vi "Main.vi"() -> ()   [LabVIEW 2021] (continued)
                w86 = T9 27 items=["刷新间隔", "波特率", "布尔1设置项", "布尔2设置项", "布尔3设置项", "布尔4设置项", "布尔5设置项", "布尔6设置项", "布尔7设置项", "布尔8设置项", "显控1设置", "显控2设置", "显控3设置", "显控4设置", "显控5设置", "显控6设置", "显控7设置", "显控8设置", "显控9设置", "显控10设置", "显控11设置", "显控12设置", "设控1设置", "设控2设置", "设控3设置", "设控4设置", "设控5设置", "设控6设置", "设控7设置", "设控8设置", "曲线1设置", "曲线2设置", "曲线3设置", "曲线4设置", "曲线5设置", "曲线6设置", "曲线7设置", "曲线8设置", "曲线9设置", "曲线10设置", "曲线11设置", "曲线12设置", "曲线13设置", "曲线14设置", "曲线15设置", "曲线16设置", "曲线17设置", "曲线18设置", "曲线19设置", "曲线20设置", "曲线21设置", "曲线22设置", "曲线23设置", "曲线24设置", "曲线25设置", "曲线26设置", "曲线27设置", "曲线28设置", "曲线29设置", "曲线30设置", "曲线31设置", "曲线32设置", "曲线33设置", "曲线34设置", "曲线35设置", "曲线36设置", "曲线37设置", "曲线38设置", "曲线39设置", "曲线40设置", "曲线41设置", "曲线42设置", "曲线43设置", "曲线44设置", "曲线45设置", "曲线46设置", "曲线47设置", "曲线48设置", "曲线49设置", "曲线50设置", "曲线51设置", "曲线52设置", "曲线53设置", "曲线54设置", "曲线55设置", "曲线56设置", "曲线57设置", "曲线58设置", "曲线59设置", "曲线60设置", "曲线61设置", "曲线62设置", "曲线63设置", "曲线64设置", "ID值", "数据模式"] ("DataInitDef")
                w87 = T9 26 items=["刷新间隔", "波特率", "布尔1设置项", "布尔2设置项", "布尔3设置项", "布尔4设置项", "布尔5设置项", "布尔6设置项", "布尔7设置项", "布尔8设置项", "显控1设置", "显控2设置", "显控3设置", "显控4设置", "显控5设置", "显控6设置", "显控7设置", "显控8设置", "显控9设置", "显控10设置", "显控11设置", "显控12设置", "设控1设置", "设控2设置", "设控3设置", "设控4设置", "设控5设置", "设控6设置", "设控7设置", "设控8设置", "曲线1设置", "曲线2设置", "曲线3设置", "曲线4设置", "曲线5设置", "曲线6设置", "曲线7设置", "曲线8设置", "曲线9设置", "曲线10设置", "曲线11设置", "曲线12设置", "曲线13设置", "曲线14设置", "曲线15设置", "曲线16设置", "曲线17设置", "曲线18设置", "曲线19设置", "曲线20设置", "曲线21设置", "曲线22设置", "曲线23设置", "曲线24设置", "曲线25设置", "曲线26设置", "曲线27设置", "曲线28设置", "曲线29设置", "曲线30设置", "曲线31设置", "曲线32设置", "曲线33设置", "曲线34设置", "曲线35设置", "曲线36设置", "曲线37设置", "曲线38设置", "曲线39设置", "曲线40设置", "曲线41设置", "曲线42设置", "曲线43设置", "曲线44设置", "曲线45设置", "曲线46设置", "曲线47设置", "曲线48设置", "曲线49设置", "曲线50设置", "曲线51设置", "曲线52设置", "曲线53设置", "曲线54设置", "曲线55设置", "曲线56设置", "曲线57设置", "曲线58设置", "曲线59设置", "曲线60设置", "曲线61设置", "曲线62设置", "曲线63设置", "曲线64设置", "ID值", "数据模式"] ("DataInitDef")
                w88 = T9 29 items=["刷新间隔", "波特率", "布尔1设置项", "布尔2设置项", "布尔3设置项", "布尔4设置项", "布尔5设置项", "布尔6设置项", "布尔7设置项", "布尔8设置项", "显控1设置", "显控2设置", "显控3设置", "显控4设置", "显控5设置", "显控6设置", "显控7设置", "显控8设置", "显控9设置", "显控10设置", "显控11设置", "显控12设置", "设控1设置", "设控2设置", "设控3设置", "设控4设置", "设控5设置", "设控6设置", "设控7设置", "设控8设置", "曲线1设置", "曲线2设置", "曲线3设置", "曲线4设置", "曲线5设置", "曲线6设置", "曲线7设置", "曲线8设置", "曲线9设置", "曲线10设置", "曲线11设置", "曲线12设置", "曲线13设置", "曲线14设置", "曲线15设置", "曲线16设置", "曲线17设置", "曲线18设置", "曲线19设置", "曲线20设置", "曲线21设置", "曲线22设置", "曲线23设置", "曲线24设置", "曲线25设置", "曲线26设置", "曲线27设置", "曲线28设置", "曲线29设置", "曲线30设置", "曲线31设置", "曲线32设置", "曲线33设置", "曲线34设置", "曲线35设置", "曲线36设置", "曲线37设置", "曲线38设置", "曲线39设置", "曲线40设置", "曲线41设置", "曲线42设置", "曲线43设置", "曲线44设置", "曲线45设置", "曲线46设置", "曲线47设置", "曲线48设置", "曲线49设置", "曲线50设置", "曲线51设置", "曲线52设置", "曲线53设置", "曲线54设置", "曲线55设置", "曲线56设置", "曲线57设置", "曲线58设置", "曲线59设置", "曲线60设置", "曲线61设置", "曲线62设置", "曲线63设置", "曲线64设置", "ID值", "数据模式"] ("DataInitDef")
                w89 = T9 24 items=["刷新间隔", "波特率", "布尔1设置项", "布尔2设置项", "布尔3设置项", "布尔4设置项", "布尔5设置项", "布尔6设置项", "布尔7设置项", "布尔8设置项", "显控1设置", "显控2设置", "显控3设置", "显控4设置", "显控5设置", "显控6设置", "显控7设置", "显控8设置", "显控9设置", "显控10设置", "显控11设置", "显控12设置", "设控1设置", "设控2设置", "设控3设置", "设控4设置", "设控5设置", "设控6设置", "设控7设置", "设控8设置", "曲线1设置", "曲线2设置", "曲线3设置", "曲线4设置", "曲线5设置", "曲线6设置", "曲线7设置", "曲线8设置", "曲线9设置", "曲线10设置", "曲线11设置", "曲线12设置", "曲线13设置", "曲线14设置", "曲线15设置", "曲线16设置", "曲线17设置", "曲线18设置", "曲线19设置", "曲线20设置", "曲线21设置", "曲线22设置", "曲线23设置", "曲线24设置", "曲线25设置", "曲线26设置", "曲线27设置", "曲线28设置", "曲线29设置", "曲线30设置", "曲线31设置", "曲线32设置", "曲线33设置", "曲线34设置", "曲线35设置", "曲线36设置", "曲线37设置", "曲线38设置", "曲线39设置", "曲线40设置", "曲线41设置", "曲线42设置", "曲线43设置", "曲线44设置", "曲线45设置", "曲线46设置", "曲线47设置", "曲线48设置", "曲线49设置", "曲线50设置", "曲线51设置", "曲线52设置", "曲线53设置", "曲线54设置", "曲线55设置", "曲线56设置", "曲线57设置", "曲线58设置", "曲线59设置", "曲线60设置", "曲线61设置", "曲线62设置", "曲线63设置", "曲线64设置", "ID值", "数据模式"] ("DataInitDef")
                w90 = T9 25 items=["刷新间隔", "波特率", "布尔1设置项", "布尔2设置项", "布尔3设置项", "布尔4设置项", "布尔5设置项", "布尔6设置项", "布尔7设置项", "布尔8设置项", "显控1设置", "显控2设置", "显控3设置", "显控4设置", "显控5设置", "显控6设置", "显控7设置", "显控8设置", "显控9设置", "显控10设置", "显控11设置", "显控12设置", "设控1设置", "设控2设置", "设控3设置", "设控4设置", "设控5设置", "设控6设置", "设控7设置", "设控8设置", "曲线1设置", "曲线2设置", "曲线3设置", "曲线4设置", "曲线5设置", "曲线6设置", "曲线7设置", "曲线8设置", "曲线9设置", "曲线10设置", "曲线11设置", "曲线12设置", "曲线13设置", "曲线14设置", "曲线15设置", "曲线16设置", "曲线17设置", "曲线18设置", "曲线19设置", "曲线20设置", "曲线21设置", "曲线22设置", "曲线23设置", "曲线24设置", "曲线25设置", "曲线26设置", "曲线27设置", "曲线28设置", "曲线29设置", "曲线30设置", "曲线31设置", "曲线32设置", "曲线33设置", "曲线34设置", "曲线35设置", "曲线36设置", "曲线37设置", "曲线38设置", "曲线39设置", "曲线40设置", "曲线41设置", "曲线42设置", "曲线43设置", "曲线44设置", "曲线45设置", "曲线46设置", "曲线47设置", "曲线48设置", "曲线49设置", "曲线50设置", "曲线51设置", "曲线52设置", "曲线53设置", "曲线54设置", "曲线55设置", "曲线56设置", "曲线57设置", "曲线58设置", "曲线59设置", "曲线60设置", "曲线61设置", "曲线62设置", "曲线63设置", "曲线64设置", "ID值", "数据模式"] ("DataInitDef")
                w91 = T9 23 items=["刷新间隔", "波特率", "布尔1设置项", "布尔2设置项", "布尔3设置项", "布尔4设置项", "布尔5设置项", "布尔6设置项", "布尔7设置项", "布尔8设置项", "显控1设置", "显控2设置", "显控3设置", "显控4设置", "显控5设置", "显控6设置", "显控7设置", "显控8设置", "显控9设置", "显控10设置", "显控11设置", "显控12设置", "设控1设置", "设控2设置", "设控3设置", "设控4设置", "设控5设置", "设控6设置", "设控7设置", "设控8设置", "曲线1设置", "曲线2设置", "曲线3设置", "曲线4设置", "曲线5设置", "曲线6设置", "曲线7设置", "曲线8设置", "曲线9设置", "曲线10设置", "曲线11设置", "曲线12设置", "曲线13设置", "曲线14设置", "曲线15设置", "曲线16设置", "曲线17设置", "曲线18设置", "曲线19设置", "曲线20设置", "曲线21设置", "曲线22设置", "曲线23设置", "曲线24设置", "曲线25设置", "曲线26设置", "曲线27设置", "曲线28设置", "曲线29设置", "曲线30设置", "曲线31设置", "曲线32设置", "曲线33设置", "曲线34设置", "曲线35设置", "曲线36设置", "曲线37设置", "曲线38设置", "曲线39设置", "曲线40设置", "曲线41设置", "曲线42设置", "曲线43设置", "曲线44设置", "曲线45设置", "曲线46设置", "曲线47设置", "曲线48设置", "曲线49设置", "曲线50设置", "曲线51设置", "曲线52设置", "曲线53设置", "曲线54设置", "曲线55设置", "曲线56设置", "曲线57设置", "曲线58设置", "曲线59设置", "曲线60设置", "曲线61设置", "曲线62设置", "曲线63设置", "曲线64设置", "ID值", "数据模式"] ("DataInitDef")
                w92 = T9 94 items=["刷新间隔", "波特率", "布尔1设置项", "布尔2设置项", "布尔3设置项", "布尔4设置项", "布尔5设置项", "布尔6设置项", "布尔7设置项", "布尔8设置项", "显控1设置", "显控2设置", "显控3设置", "显控4设置", "显控5设置", "显控6设置", "显控7设置", "显控8设置", "显控9设置", "显控10设置", "显控11设置", "显控12设置", "设控1设置", "设控2设置", "设控3设置", "设控4设置", "设控5设置", "设控6设置", "设控7设置", "设控8设置", "曲线1设置", "曲线2设置", "曲线3设置", "曲线4设置", "曲线5设置", "曲线6设置", "曲线7设置", "曲线8设置", "曲线9设置", "曲线10设置", "曲线11设置", "曲线12设置", "曲线13设置", "曲线14设置", "曲线15设置", "曲线16设置", "曲线17设置", "曲线18设置", "曲线19设置", "曲线20设置", "曲线21设置", "曲线22设置", "曲线23设置", "曲线24设置", "曲线25设置", "曲线26设置", "曲线27设置", "曲线28设置", "曲线29设置", "曲线30设置", "曲线31设置", "曲线32设置", "曲线33设置", "曲线34设置", "曲线35设置", "曲线36设置", "曲线37设置", "曲线38设置", "曲线39设置", "曲线40设置", "曲线41设置", "曲线42设置", "曲线43设置", "曲线44设置", "曲线45设置", "曲线46设置", "曲线47设置", "曲线48设置", "曲线49设置", "曲线50设置", "曲线51设置", "曲线52设置", "曲线53设置", "曲线54设置", "曲线55设置", "曲线56设置", "曲线57设置", "曲线58设置", "曲线59设置", "曲线60设置", "曲线61设置", "曲线62设置", "曲线63设置", "曲线64设置", "ID值", "数据模式"] ("DataInitDef")
                w93 = T9 22 items=["刷新间隔", "波特率", "布尔1设置项", "布尔2设置项", "布尔3设置项", "布尔4设置项", "布尔5设置项", "布尔6设置项", "布尔7设置项", "布尔8设置项", "显控1设置", "显控2设置", "显控3设置", "显控4设置", "显控5设置", "显控6设置", "显控7设置", "显控8设置", "显控9设置", "显控10设置", "显控11设置", "显控12设置", "设控1设置", "设控2设置", "设控3设置", "设控4设置", "设控5设置", "设控6设置", "设控7设置", "设控8设置", "曲线1设置", "曲线2设置", "曲线3设置", "曲线4设置", "曲线5设置", "曲线6设置", "曲线7设置", "曲线8设置", "曲线9设置", "曲线10设置", "曲线11设置", "曲线12设置", "曲线13设置", "曲线14设置", "曲线15设置", "曲线16设置", "曲线17设置", "曲线18设置", "曲线19设置", "曲线20设置", "曲线21设置", "曲线22设置", "曲线23设置", "曲线24设置", "曲线25设置", "曲线26设置", "曲线27设置", "曲线28设置", "曲线29设置", "曲线30设置", "曲线31设置", "曲线32设置", "曲线33设置", "曲线34设置", "曲线35设置", "曲线36设置", "曲线37设置", "曲线38设置", "曲线39设置", "曲线40设置", "曲线41设置", "曲线42设置", "曲线43设置", "曲线44设置", "曲线45设置", "曲线46设置", "曲线47设置", "曲线48设置", "曲线49设置", "曲线50设置", "曲线51设置", "曲线52设置", "曲线53设置", "曲线54设置", "曲线55设置", "曲线56设置", "曲线57设置", "曲线58设置", "曲线59设置", "曲线60设置", "曲线61设置", "曲线62设置", "曲线63设置", "曲线64设置", "ID值", "数据模式"] ("DataInitDef")
                w103 = 0 ("禁用的索引 (列)")
                w102 = 0 ("禁用的索引 (列)")
                n54 = local read "控件配置文件"() -> (w96:string[][])
                n55 = local read "控件配置文件"() -> (w108:string[][])
                n56 = Index Array(array=w96, index (row)=w93, index (col)=w102) -> (element=w111:string)
                n57 = Index Array(array=w96, index (row)=w91, index (col)=w102) -> (element=w110:string)
                n58 = Index Array(array=w96, index (row)=w90, index (col)=w102) -> (element=w109:string)
                n59 = Index Array(array=w96, index (row)=w89, index (col)=w102) -> (element=w112:string)
                n60 = Index Array(array=w108, index (row)=w88, index (col)=w103) -> (element=w107:string)
                n61 = Index Array(array=w108, index (row)=w87, index (col)=w103) -> (element=w105:string)
                n62 = Index Array(array=w108, index (row)=w86, index (col)=w103) -> (element=w106:string)
                n63 = Index Array(array=w108, index (row)=w85, index (col)=w103) -> (element=w104:string)
                n64 = Index Array(array=w96, index (row)=w92, index (col)=1 ("禁用的索引 (列)")) -> (element=w100:string)
                n65 = property on="设控1" class="Str"("Caption.Text"=w111) -> ()  [unwired: 2 in, 2 out]
                n66 = property on="设控2" class="Str"("Caption.Text"=w110) -> ()  [unwired: 2 in, 2 out]
                n67 = property on="设控4" class="Str"("Caption.Text"=w109) -> ()  [unwired: 2 in, 2 out]
                n68 = property on="设控3" class="Str"("Caption.Text"=w112) -> ()  [unwired: 2 in, 2 out]
                n69 = property on="设控8" class="Str"("Caption.Text"=w107) -> ()  [unwired: 2 in, 2 out]
                n70 = property on="设控5" class="Str"("Caption.Text"=w105) -> ()  [unwired: 2 in, 2 out]
                n71 = property on="设控6" class="Str"("Caption.Text"=w106) -> ()  [unwired: 2 in, 2 out]
                n72 = property on="设控7" class="Str"("Caption.Text"=w104) -> ()  [unwired: 2 in, 2 out]
                n73 = Hexadecimal String To Number(string=w100) -> (number=w99:u32)  [unwired: 2 in, 1 out]
                n74 = local write "ID"(w99) -> ()
                n75 = Index Array(array=w96, index (row)=w84, index (col)=1 ("禁用的索引 (列)")) -> (element=w97:string)
                n76 = Hexadecimal String To Number(string=w97) -> (number=w95:u32)  [unwired: 2 in, 1 out]
                n77 = Not Equal To 0?(x=w95) -> (x != 0?=w94:bool)
                n78 = local write "数据模式"(w94) -> ()
              }
              frame #3 {
                w113 = T9 9 items=["刷新间隔", "波特率", "布尔1设置项", "布尔2设置项", "布尔3设置项", "布尔4设置项", "布尔5设置项", "布尔6设置项", "布尔7设置项", "布尔8设置项", "显控1设置", "显控2设置", "显控3设置", "显控4设置", "显控5设置", "显控6设置", "显控7设置", "显控8设置", "显控9设置", "显控10设置", "显控11设置", "显控12设置", "设控1设置", "设控2设置", "设控3设置", "设控4设置", "设控5设置", "设控6设置", "设控7设置", "设控8设置", "曲线1设置", "曲线2设置", "曲线3设置", "曲线4设置", "曲线5设置", "曲线6设置", "曲线7设置", "曲线8设置", "曲线9设置", "曲线10设置", "曲线11设置", "曲线12设置", "曲线13设置", "曲线14设置", "曲线15设置", "曲线16设置", "曲线17设置", "曲线18设置", "曲线19设置", "曲线20设置", "曲线21设置", "曲线22设置", "曲线23设置", "曲线24设置", "曲线25设置", "曲线26设置", "曲线27设置", "曲线28设置", "曲线29设置", "曲线30设置", "曲线31设置", "曲线32设置", "曲线33设置", "曲线34设置", "曲线35设置", "曲线36设置", "曲线37设置", "曲线38设置", "曲线39设置", "曲线40设置", "曲线41设置", "曲线42设置", "曲线43设置", "曲线44设置", "曲线45设置", "曲线46设置", "曲线47设置", "曲线48设置", "曲线49设置", "曲线50设置", "曲线51设置", "曲线52设置", "曲线53设置", "曲线54设置", "曲线55设置", "曲线56设置", "曲线57设置", "曲线58设置", "曲线59设置", "曲线60设置", "曲线61设置", "曲线62设置", "曲线63设置", "曲线64设置", "ID值", "数据模式"] ("DataInitDef")
                w114 = T9 8 items=["刷新间隔", "波特率", "布尔1设置项", "布尔2设置项", "布尔3设置项", "布尔4设置项", "布尔5设置项", "布尔6设置项", "布尔7设置项", "布尔8设置项", "显控1设置", "显控2设置", "显控3设置", "显控4设置", "显控5设置", "显控6设置", "显控7设置", "显控8设置", "显控9设置", "显控10设置", "显控11设置", "显控12设置", "设控1设置", "设控2设置", "设控3设置", "设控4设置", "设控5设置", "设控6设置", "设控7设置", "设控8设置", "曲线1设置", "曲线2设置", "曲线3设置", "曲线4设置", "曲线5设置", "曲线6设置", "曲线7设置", "曲线8设置", "曲线9设置", "曲线10设置", "曲线11设置", "曲线12设置", "曲线13设置", "曲线14设置", "曲线15设置", "曲线16设置", "曲线17设置", "曲线18设置", "曲线19设置", "曲线20设置", "曲线21设置", "曲线22设置", "曲线23设置", "曲线24设置", "曲线25设置", "曲线26设置", "曲线27设置", "曲线28设置", "曲线29设置", "曲线30设置", "曲线31设置", "曲线32设置", "曲线33设置", "曲线34设置", "曲线35设置", "曲线36设置", "曲线37设置", "曲线38设置", "曲线39设置", "曲线40设置", "曲线41设置", "曲线42设置", "曲线43设置", "曲线44设置", "曲线45设置", "曲线46设置", "曲线47设置", "曲线48设置", "曲线49设置", "曲线50设置", "曲线51设置", "曲线52设置", "曲线53设置", "曲线54设置", "曲线55设置", "曲线56设置", "曲线57设置", "曲线58设置", "曲线59设置", "曲线60设置", "曲线61设置", "曲线62设置", "曲线63设置", "曲线64设置", "ID值", "数据模式"] ("DataInitDef")
                w115 = T9 7 items=["刷新间隔", "波特率", "布尔1设置项", "布尔2设置项", "布尔3设置项", "布尔4设置项", "布尔5设置项", "布尔6设置项", "布尔7设置项", "布尔8设置项", "显控1设置", "显控2设置", "显控3设置", "显控4设置", "显控5设置", "显控6设置", "显控7设置", "显控8设置", "显控9设置", "显控10设置", "显控11设置", "显控12设置", "设控1设置", "设控2设置", "设控3设置", "设控4设置", "设控5设置", "设控6设置", "设控7设置", "设控8设置", "曲线1设置", "曲线2设置", "曲线3设置", "曲线4设置", "曲线5设置", "曲线6设置", "曲线7设置", "曲线8设置", "曲线9设置", "曲线10设置", "曲线11设置", "曲线12设置", "曲线13设置", "曲线14设置", "曲线15设置", "曲线16设置", "曲线17设置", "曲线18设置", "曲线19设置", "曲线20设置", "曲线21设置", "曲线22设置", "曲线23设置", "曲线24设置", "曲线25设置", "曲线26设置", "曲线27设置", "曲线28设置", "曲线29设置", "曲线30设置", "曲线31设置", "曲线32设置", "曲线33设置", "曲线34设置", "曲线35设置", "曲线36设置", "曲线37设置", "曲线38设置", "曲线39设置", "曲线40设置", "曲线41设置", "曲线42设置", "曲线43设置", "曲线44设置", "曲线45设置", "曲线46设置", "曲线47设置", "曲线48设置", "曲线49设置", "曲线50设置", "曲线51设置", "曲线52设置", "曲线53设置", "曲线54设置", "曲线55设置", "曲线56设置", "曲线57设置", "曲线58设置", "曲线59设置", "曲线60设置", "曲线61设置", "曲线62设置", "曲线63设置", "曲线64设置", "ID值", "数据模式"] ("DataInitDef")
                w116 = 0 ("禁用的索引 (列)")
                n79 = local read "控件配置文件"() -> (w117:string[][])
                n80 = Index Array(array=w117, index (row)=w115, index (col)=w116) -> (element=w118:string)
                n81 = Index Array(array=w117, index (row)=w114, index (col)=w116) -> (element=w119:string)
                n82 = Index Array(array=w117, index (row)=w113, index (col)=w116) -> (element=w120:string)
                n83 = property on="布尔 6" class="Bool (严格)"("Caption.Text"=w118) -> ()  [unwired: 2 in, 2 out]
                n84 = property on="布尔 7" class="Bool (严格)"("Caption.Text"=w119) -> ()  [unwired: 2 in, 2 out]
                n85 = property on="布尔 8" class="Bool (严格)"("Caption.Text"=w120) -> ()  [unwired: 2 in, 2 out]
              }
              frame #4 {
                n86 = stacked-sequence {
                  seq-local: [w121 _ _] -> [_ w131 w140]
                  frame #0 {
                    n87 = call <vilib>:"Application Directory.vi"() -> ("Application Directory"=w127:path)
                    n88 = Build Path(base path=w127, name or relative path="Config\\DATA.txt" ("名称或相对路径")) -> (appended path=w128:path)
                    n89 = Open/Create/Replace File(file path (use dialog)=w128) -> (refnum out=w126:refnum<file>, error out=w125:errorcluster)  [unwired: 5 in, 1 out]
                    n90 = Read from Text File "读取文本文件"(file (use dialog)=w126, error in=w125) -> (refnum out=w129:refnum<file>, text=w124:string, error out=w130:errorcluster)  [unwired: 2 in, 1 out]
                    n91 = Close File(refnum=w129, error in=w130) -> ()  [unwired: 2 out]
                    n92 = Spreadsheet String To Array(format string="%s" ("格式字符串"), spreadsheet string=w124, array type (2D Dbl)=w124) -> (array=w121:string[][])  [unwired: 1 in]
                  }
                  frame #1 {
                    n93 = Index Array(array=w131, index (row)=0 ("索引 (行)")) -> (element=w133:string[])  [unwired: 1 in]
                    n94 = property on="表格" class="Tbl (严格)"("Column Headers[]"=w133) -> ()  [unwired: 2 in, 2 out]
                  }
                  frame #2 {
                    # "显示表格数据初始化"
                    n95 = Delete From Array "删除数组元素"(array=w140, index (row)=0 ("索引 (行)")) -> (array with subset deleted=w138:string[][])  [unwired: 2 in, 1 out]
                    n96 = Array Size(array=w138) -> (size(s)=w139:i32[])
                    n97 = for "For循环" {
                      tunnel: w138 -> [w149] mode=indexing
                      tunnel: [w143] -> w137 mode=indexing
                      n98 = Index Array(array=w149, index=1 ("索引")) -> (element=w148:string)
                      n99 = Index Array(array=w149, index=7 ("索引")) -> (element=w147:string)
                      n100 = Decimal String To Number(string=w147) -> (number=w144:i32)  [unwired: 2 in, 1 out]
                      n101 = Decimal String To Number(string=w148) -> (number=w146:i32)  [unwired: 2 in, 1 out]
                      n102 = Build Array(w146, u32 0 ("元素"), w144) -> (w143:u32[])
                    }
                    n103 = property on="表格" class="Tbl (严格)"("Value"=w138) -> ()  [unwired: 2 in, 2 out]
                    n104 = Index Array(array=w139, index=0 ("索引")) -> (element=w135:i32)
                    n105 = Decrement(x=w135) -> (x-1=w134:i32)
                    "当前显示表格总行数" <- w134
                    n106 = Delete From Array "删除数组元素"(array=w137, index (row)=w134) -> (array with subset deleted=→"CANBURF":u32[][])  [unwired: 2 in, 1 out]
                  }
                }
              }
            }
          }
          frame "Process" {
            n107 = property on="表格" class="Tbl (严格)"() -> ("Selection Start"=w156:T1)  [unwired: 2 in, 2 out]
            n108 = Unbundle By Name(w156) -> ("Column"=w154:i32, "Row"=w153:i32)
            n109 = property on="表格" class="Tbl (严格)"() -> ("Value"=w162:string[][])  [unwired: 2 in, 2 out]
            n110 = Index Array(array=w162, index (row)=w153, index (col)=0 ("禁用的索引 (列)")) -> (element=w165:string)
            n111 = Index Array(array=w162, index (row)=w153, index (col)=3 ("禁用的索引 (列)")) -> (element=w160:string)
            n112 = local read "选择区域起始"() -> (w157:T1)
            n113 = event shown="[2] \"表格\": 值改变" {
              selector: _ -> [_ _ _ _]
              dyn-events: _ -> [_ _ _ _]
              timeout: 0 -> [_ _ _ _]
              tunnel: w153 -> [_ w175 w210 w253]
              tunnel: "设置" -> [_ w176 _ w254]
              tunnel: w154 -> [_ _ w207 _]
              event Timeout {
                n114 = event-data() -> ()  [unwired: 1 in, 3 out]
              }
              event "确定按钮": Value Change {
                # "本结构实现参数设置"
                n115 = event-data() -> ()  [unwired: 1 in, 3 out]
                n116 = Two Button Dialog(message="确定更改" ("消息"), 1:"否" ("F按钮名称（“取消”）"), 2:"是" ("T按钮名称（“确定”）")) -> (T button?=w174:bool)
                n117 = case shown="真" w174 {
                  tunnel: w176 -> [_ w196]
                  tunnel: w175 -> [_ w183]
                  frame False {
                  }
                  frame True {
                    # "捆绑发送数据时，地址在前，数据在后。"
                    n118 = Fract/Exp String To Number(string=w196) -> (number=w193:dbl)  [unwired: 3 in, 1 out]
                    n119 = property on="表格" class="Tbl (严格)"() -> ("Value"=w184:string[][])  [unwired: 2 in, 2 out]
                    n120 = invoke on="表格" class="Tbl (严格)" method="Set Cell Value"("X Index"=3 ("X索引"), "Y Index"=w183, "Value"=w196) -> ()  [unwired: 3 in, 6 out]
                    n121 = Index Array(array=w184, index (row)=w183, index (col)=1 ("禁用的索引 (列)")) -> (element=w188:string)
                    n122 = Index Array(array=w184, index (row)=w183, index (col)=5 ("禁用的索引 (行)")) -> (element=w195:string)
                    n123 = Decimal String To Number(string=w188) -> (number=w187:i32)  [unwired: 2 in, 1 out]
                    n124 = Fract/Exp String To Number(string=w195) -> (number=w192:dbl)  [unwired: 3 in, 1 out]
                    n125 = Greater Than 0?(x=w192) -> (x > 0?=w194:bool)
                    n126 = case shown="真" w194 {
                      tunnel: w193 -> [w199 w203]
                      tunnel: w192 -> [_ w202]
                      tunnel: [w198 w200] -> w191
                      frame False {
                        n127 = To Quad Integer(1:w199) -> (0:w198:i64)
                      }
                      frame True {
                        n128 = Divide(x=w203, y=w202) -> (x/y=w201:dbl)
                        n129 = To Quad Integer(1:w201) -> (0:w200:i64)
                      }
                    }
                    n130 = To Unsigned Word Integer(number=w187) -> (unsigned 16bit integer=w186:u16)
                    n131 = Index Array(array=w184, index (row)=w183, index (col)=7 ("禁用的索引 (列)")) -> (element=w181:string)
                    n132 = Hexadecimal String To Number(string=w181) -> (number=w180:u32)  [unwired: 2 in, 1 out]
                    n133 = Bundle(w186, w191, "Row"=w183, w180) -> (w185:cluster{u16, i64, "Row":i32, u32})  [unwired: 1 in]
                    n134 = property on="要发送的数据" class="Clust (严格)"("Val(Sgnl)"=w185) -> ()  [unwired: 2 in, 2 out]
                  }
                }
              }
              event "表格": Value Change {
                # "本结构实现参数设置"
                n135 = event-data() -> ("OldVal"=w204:string[][], "NewVal"=w211:string[][])  [unwired: 1 in, 2 out]
                n136 = Equal?(x=w207, y=3) -> (x = y?=w205:bool)
                n137 = case shown="假" w205 {
                  tunnel: [FALSE ("T button?") w215] -> w212
                  tunnel: w204 -> [w214 _]
                  frame False {
                    n138 = property on="表格" class="Tbl (严格)"("Value"=w214) -> ()  [unwired: 2 in, 2 out]
                  }
                  frame True {
                    n139 = Two Button Dialog(message="确定更改" ("消息"), 1:"否" ("F按钮名称（“取消”）"), 2:"是" ("T按钮名称（“确定”）")) -> (T button?=w215:bool)
                  }
                }
                n140 = Index Array(array=w211, index (row)=w210, index (col)=3 ("禁用的索引 (列)")) -> (element=w209:string)
                n141 = case shown="真" w212 {
                  tunnel: w209 -> [_ w235]
                  tunnel: w210 -> [_ w222]
                  frame False {
                  }
                  frame True {
                    # "捆绑发送数据时，地址在前，数据在后。"
                    n142 = Fract/Exp String To Number(string=w235) -> (number=w232:dbl)  [unwired: 3 in, 1 out]
                    n143 = property on="表格" class="Tbl (严格)"() -> ("Value"=w223:string[][])  [unwired: 2 in, 2 out]
                    n144 = invoke on="表格" class="Tbl (严格)" method="Set Cell Value"("X Index"=3 ("X索引"), "Y Index"=w222, "Value"=w235) -> ()  [unwired: 3 in, 6 out]
                    n145 = Index Array(array=w223, index (row)=w222, index (col)=1 ("禁用的索引 (列)")) -> (element=w227:string)
                    n146 = Index Array(array=w223, index (row)=w222, index (col)=5 ("禁用的索引 (行)")) -> (element=w234:string)
                    n147 = Decimal String To Number(string=w227) -> (number=w226:i32)  [unwired: 2 in, 1 out]
                    n148 = Fract/Exp String To Number(string=w234) -> (number=w231:dbl)  [unwired: 3 in, 1 out]
                    n149 = Greater Than 0?(x=w231) -> (x > 0?=w233:bool)
                    n150 = case shown="真" w233 {
                      tunnel: w232 -> [w238 w242]
                      tunnel: w231 -> [_ w241]
                      tunnel: [w237 w239] -> w230
                      frame False {
                        n151 = To Quad Integer(1:w238) -> (0:w237:i64)
                      }
                      frame True {
                        n152 = Divide(x=w242, y=w241) -> (x/y=w240:dbl)
                        n153 = To Quad Integer(1:w240) -> (0:w239:i64)
                      }
                    }
                    n154 = To Unsigned Word Integer(number=w226) -> (unsigned 16bit integer=w225:u16)
                    n155 = Index Array(array=w223, index (row)=w222, index (col)=7 ("禁用的索引 (列)")) -> (element=w220:string)
                    n156 = Hexadecimal String To Number(string=w220) -> (number=w219:u32)  [unwired: 2 in, 1 out]
                    n157 = Bundle(w225, w230, "Row"=w222, w219) -> (w224:cluster{u16, i64, "Row":i32, u32})  [unwired: 1 in]
                    n158 = property on="要发送的数据" class="Clust (严格)"("Val(Sgnl)"=w224) -> ()  [unwired: 2 in, 2 out]
                  }
                }
              }
              event Key Down {
                n159 = event-data() -> ("VKey"=w247:T7, "FocusObj"=w251:refnum<vi>)  [unwired: 1 in, 4 out]
                n160 = property on="设置" class="Str"() -> ("Text.Owner"=w250:refnum<vi>)  [unwired: 2 in, 2 out]
                n161 = Equal?(x=w247, y=eventvkey."Enter") -> (x = y?=w244:bool)
                n162 = Equal?(x=w251, y=w250) -> (x = y?=w248:bool)
                n163 = Equal?(x=w247, y=eventvkey."Return") -> (x = y?=w245:bool)
                n164 = Or(x=w245, y=w244) -> (x .or. y?=w243:bool)
                n165 = And(x=w243, y=w248) -> (x .and. y?=w249:bool)
                n166 = case shown="真" w249 {
                  tunnel: w254 -> [_ w256]
                  tunnel: w253 -> [_ w255]
                  frame False {
                  }
                  frame True {
                    n167 = Two Button Dialog(message="确定更改" ("消息"), 1:"否" ("F按钮名称（“取消”）"), 2:"是" ("T按钮名称（“确定”）")) -> (T button?=w257:bool)
                    n168 = case shown="真" w257 {
                      tunnel: w256 -> [_ w272]
                      tunnel: w255 -> [_ w262]
                      frame False {
                      }
                      frame True {
                        n169 = property on="表格" class="Tbl (严格)"() -> ("Value"=w263:string[][])  [unwired: 2 in, 2 out]
                        n170 = Fract/Exp String To Number(string=w272) -> (number=w271:dbl)  [unwired: 3 in, 1 out]
                        n171 = invoke on="表格" class="Tbl (严格)" method="Set Cell Value"("X Index"=3 ("X索引"), "Y Index"=w262, "Value"=w272) -> ()  [unwired: 3 in, 6 out]
                        n172 = Index Array(array=w263, index (row)=w262, index (col)=1 ("禁用的索引 (列)")) -> (element=w270:string)
                        n173 = Index Array(array=w263, index (row)=w262, index (col)=5 ("禁用的索引 (行)")) -> (element=w277:string)
                        n174 = Decimal String To Number(string=w270) -> (number=w268:i32)  [unwired: 2 in, 1 out]
                        n175 = Fract/Exp String To Number(string=w277) -> (number=w275:dbl)  [unwired: 3 in, 1 out]
                        n176 = Greater Than 0?(x=w275) -> (x > 0?=w276:bool)
                        n177 = To Unsigned Word Integer(number=w268) -> (unsigned 16bit integer=w267:u16)
                        n178 = case shown="真" w276 {
                          tunnel: w271 -> [w280 w284]
                          tunnel: w275 -> [_ w283]
                          tunnel: [w279 w281] -> w269
                          frame False {
                            n179 = To Quad Integer(1:w280) -> (0:w279:i64)
                          }
                          frame True {
                            n180 = Divide(x=w284, y=w283) -> (x/y=w282:dbl)
                            n181 = To Quad Integer(1:w282) -> (0:w281:i64)
                          }
                        }
                        n182 = Index Array(array=w263, index (row)=w262, index (col)=7 ("禁用的索引 (列)")) -> (element=w264:string)
                        n183 = Hexadecimal String To Number(string=w264) -> (offset past number=w261:i32)  [unwired: 2 in, 1 out]
                        n184 = Bundle(w267, w269, "Row"=w262, "offset past number"=w261) -> (w266:T10)  [unwired: 1 in]
                        n185 = property on="要发送的数据" class="Clust (严格)"("Val(Sgnl)"=w266) -> ()  [unwired: 2 in, 2 out]
                      }
                    }
                  }
                }
              }
            }
            n186 = String Subset(string=w165, length (rest)=28 ("长度（剩余）")) -> (substring=w164:string)  [unwired: 1 in]
            n187 = property on="设置" class="Str"("Caption.Text"=w164) -> ()  [unwired: 2 in, 2 out]
            n188 = Unbundle By Name(w157) -> ("Row"=w152:i32)
            n189 = Not Equal?(x=w153, y=w152) -> (x != y?=w159:bool)
            n190 = case shown="真" w159 {
              tunnel: w160 -> [_ w173]
              frame False {
              }
              frame True {
                n191 = property on="设置" class="Str"("Text.Text"=w173) -> ()  [unwired: 2 in, 2 out]
                n192 = property on="表格" class="Tbl (严格)"() -> ("Selection Start"=→"选择区域起始":T1)  [unwired: 2 in, 2 out]
              }
            }
            n193 = event shown="[1] \"选择参数表\": 值改变" {
              selector: _ -> [_ _]
              dyn-events: _ -> [_ _]
              timeout: 0 -> [_ _]
              tunnel: [FALSE TRUE] -> w171
              event Timeout {
                n194 = event-data() -> ()  [unwired: 1 in, 3 out]
              }
              event "选择参数表": Value Change {
                n195 = event-data() -> ()  [unwired: 1 in, 1 out]
              }
            }
            n196 = Select(t=ProcessState."Start" ("ProcessState"), s=w171, f=ProcessState."Process" ("ProcessState")) -> (s? t:f=w169:T2)
          }
          frame "Exit" {
            # "信号处理。信号处理引擎本身也是一个带退出的状态机"
          }
        }
      }
      frame #1 {
        n197 = stacked-sequence {
          frame #0 {
            # "布尔状态更新处理代码"
            n198 = event shown="[0] 超时" {
              selector: _ -> [_ _ _ _ _ _ _ _ _ _ _ _ _ _ _ _ _]
              dyn-events: _ -> [_ _ _ _ _ _ _ _ _ _ _ _ _ _ _ _ _]
              timeout: 0 -> [_ _ _ _ _ _ _ _ _ _ _ _ _ _ _ _ _]
              event Timeout {
                n199 = event-data() -> ()  [unwired: 1 in, 3 out]
                n200 = local read "延时更新布尔状态"() -> (w289:i16)
                n201 = Increment(x=w289) -> (x+1=w290:i16)
                n202 = Greater?(x=w289, y=i16 8) -> (0:w291:bool)
                n203 = case shown="真" w291 {
                  tunnel: w290 -> [w293 _]
                  frame False {
                    n204 = local write "延时更新布尔状态"(w293) -> ()
                  }
                  frame True {
                    w300 = T9 9 items=["刷新间隔", "波特率", "布尔1设置项", "布尔2设置项", "布尔3设置项", "布尔4设置项", "布尔5设置项", "布尔6设置项", "布尔7设置项", "布尔8设置项", "显控1设置", "显控2设置", "显控3设置", "显控4设置", "显控5设置", "显控6设置", "显控7设置", "显控8设置", "显控9设置", "显控10设置", "显控11设置", "显控12设置", "设控1设置", "设控2设置", "设控3设置", "设控4设置", "设控5设置", "设控6设置", "设控7设置", "设控8设置", "曲线1设置", "曲线2设置", "曲线3设置", "曲线4设置", "曲线5设置", "曲线6设置", "曲线7设置", "曲线8设置", "曲线9设置", "曲线10设置", "曲线11设置", "曲线12设置", "曲线13设置", "曲线14设置", "曲线15设置", "曲线16设置", "曲线17设置", "曲线18设置", "曲线19设置", "曲线20设置", "曲线21设置", "曲线22设置", "曲线23设置", "曲线24设置", "曲线25设置", "曲线26设置", "曲线27设置", "曲线28设置", "曲线29设置", "曲线30设置", "曲线31设置", "曲线32设置", "曲线33设置", "曲线34设置", "曲线35设置", "曲线36设置", "曲线37设置", "曲线38设置", "曲线39设置", "曲线40设置", "曲线41设置", "曲线42设置", "曲线43设置", "曲线44设置", "曲线45设置", "曲线46设置", "曲线47设置", "曲线48设置", "曲线49设置", "曲线50设置", "曲线51设置", "曲线52设置", "曲线53设置", "曲线54设置", "曲线55设置", "曲线56设置", "曲线57设置", "曲线58设置", "曲线59设置", "曲线60设置", "曲线61设置", "曲线62设置", "曲线63设置", "曲线64设置", "ID值", "数据模式"] ("DataInitDef")
                    w301 = T9 8 items=["刷新间隔", "波特率", "布尔1设置项", "布尔2设置项", "布尔3设置项", "布尔4设置项", "布尔5设置项", "布尔6设置项", "布尔7设置项", "布尔8设置项", "显控1设置", "显控2设置", "显控3设置", "显控4设置", "显控5设置", "显控6设置", "显控7设置", "显控8设置", "显控9设置", "显控10设置", "显控11设置", "显控12设置", "设控1设置", "设控2设置", "设控3设置", "设控4设置", "设控5设置", "设控6设置", "设控7设置", "设控8设置", "曲线1设置", "曲线2设置", "曲线3设置", "曲线4设置", "曲线5设置", "曲线6设置", "曲线7设置", "曲线8设置", "曲线9设置", "曲线10设置", "曲线11设置", "曲线12设置", "曲线13设置", "曲线14设置", "曲线15设置", "曲线16设置", "曲线17设置", "曲线18设置", "曲线19设置", "曲线20设置", "曲线21设置", "曲线22设置", "曲线23设置", "曲线24设置", "曲线25设置", "曲线26设置", "曲线27设置", "曲线28设置", "曲线29设置", "曲线30设置", "曲线31设置", "曲线32设置", "曲线33设置", "曲线34设置", "曲线35设置", "曲线36设置", "曲线37设置", "曲线38设置", "曲线39设置", "曲线40设置", "曲线41设置", "曲线42设置", "曲线43设置", "曲线44设置", "曲线45设置", "曲线46设置", "曲线47设置", "曲线48设置", "曲线49设置", "曲线50设置", "曲线51设置", "曲线52设置", "曲线53设置", "曲线54设置", "曲线55设置", "曲线56设置", "曲线57设置", "曲线58设置", "曲线59设置", "曲线60设置", "曲线61设置", "曲线62设置", "曲线63设置", "曲线64设置", "ID值", "数据模式"] ("DataInitDef")
                    w310 = T9 7 items=["刷新间隔", "波特率", "布尔1设置项", "布尔2设置项", "布尔3设置项", "布尔4设置项", "布尔5设置项", "布尔6设置项", "布尔7设置项", "布尔8设置项", "显控1设置", "显控2设置", "显控3设置", "显控4设置", "显控5设置", "显控6设置", "显控7设置", "显控8设置", "显控9设置", "显控10设置", "显控11设置", "显控12设置", "设控1设置", "设控2设置", "设控3设置", "设控4设置", "设控5设置", "设控6设置", "设控7设置", "设控8设置", "曲线1设置", "曲线2设置", "曲线3设置", "曲线4设置", "曲线5设置", "曲线6设置", "曲线7设置", "曲线8设置", "曲线9设置", "曲线10设置", "曲线11设置", "曲线12设置", "曲线13设置", "曲线14设置", "曲线15设置", "曲线16设置", "曲线17设置", "曲线18设置", "曲线19设置", "曲线20设置", "曲线21设置", "曲线22设置", "曲线23设置", "曲线24设置", "曲线25设置", "曲线26设置", "曲线27设置", "曲线28设置", "曲线29设置", "曲线30设置", "曲线31设置", "曲线32设置", "曲线33设置", "曲线34设置", "曲线35设置", "曲线36设置", "曲线37设置", "曲线38设置", "曲线39设置", "曲线40设置", "曲线41设置", "曲线42设置", "曲线43设置", "曲线44设置", "曲线45设置", "曲线46设置", "曲线47设置", "曲线48设置", "曲线49设置", "曲线50设置", "曲线51设置", "曲线52设置", "曲线53设置", "曲线54设置", "曲线55设置", "曲线56设置", "曲线57设置", "曲线58设置", "曲线59设置", "曲线60设置", "曲线61设置", "曲线62设置", "曲线63设置", "曲线64设置", "ID值", "数据模式"] ("DataInitDef")
                    w326 = T9 6 items=["刷新间隔", "波特率", "布尔1设置项", "布尔2设置项", "布尔3设置项", "布尔4设置项", "布尔5设置项", "布尔6设置项", "布尔7设置项", "布尔8设置项", "显控1设置", "显控2设置", "显控3设置", "显控4设置", "显控5设置", "显控6设置", "显控7设置", "显控8设置", "显控9设置", "显控10设置", "显控11设置", "显控12设置", "设控1设置", "设控2设置", "设控3设置", "设控4设置", "设控5设置", "设控6设置", "设控7设置", "设控8设置", "曲线1设置", "曲线2设置", "曲线3设置", "曲线4设置", "曲线5设置", "曲线6设置", "曲线7设置", "曲线8设置", "曲线9设置", "曲线10设置", "曲线11设置", "曲线12设置", "曲线13设置", "曲线14设置", "曲线15设置", "曲线16设置", "曲线17设置", "曲线18设置", "曲线19设置", "曲线20设置", "曲线21设置", "曲线22设置", "曲线23设置", "曲线24设置", "曲线25设置", "曲线26设置", "曲线27设置", "曲线28设置", "曲线29设置", "曲线30设置", "曲线31设置", "曲线32设置", "曲线33设置", "曲线34设置", "曲线35设置", "曲线36设置", "曲线37设置", "曲线38设置", "曲线39设置", "曲线40设置", "曲线41设置", "曲线42设置", "曲线43设置", "曲线44设置", "曲线45设置", "曲线46设置", "曲线47设置", "曲线48设置", "曲线49设置", "曲线50设置", "曲线51设置", "曲线52设置", "曲线53设置", "曲线54设置", "曲线55设置", "曲线56设置", "曲线57设置", "曲线58设置", "曲线59设置", "曲线60设置", "曲线61设置", "曲线62设置", "曲线63设置", "曲线64设置", "ID值", "数据模式"] ("DataInitDef")
                    w327 = T9 5 items=["刷新间隔", "波特率", "布尔1设置项", "布尔2设置项", "布尔3设置项", "布尔4设置项", "布尔5设置项", "布尔6设置项", "布尔7设置项", "布尔8设置项", "显控1设置", "显控2设置", "显控3设置", "显控4设置", "显控5设置", "显控6设置", "显控7设置", "显控8设置", "显控9设置", "显控10设置", "显控11设置", "显控12设置", "设控1设置", "设控2设置", "设控3设置", "设控4设置", "设控5设置", "设控6设置", "设控7设置", "设控8设置", "曲线1设置", "曲线2设置", "曲线3设置", "曲线4设置", "曲线5设置", "曲线6设置", "曲线7设置", "曲线8设置", "曲线9设置", "曲线10设置", "曲线11设置", "曲线12设置", "曲线13设置", "曲线14设置", "曲线15设置", "曲线16设置", "曲线17设置", "曲线18设置", "曲线19设置", "曲线20设置", "曲线21设置", "曲线22设置", "曲线23设置", "曲线24设置", "曲线25设置", "曲线26设置", "曲线27设置", "曲线28设置", "曲线29设置", "曲线30设置", "曲线31设置", "曲线32设置", "曲线33设置", "曲线34设置", "曲线35设置", "曲线36设置", "曲线37设置", "曲线38设置", "曲线39设置", "曲线40设置", "曲线41设置", "曲线42设置", "曲线43设置", "曲线44设置", "曲线45设置", "曲线46设置", "曲线47设置", "曲线48设置", "曲线49设置", "曲线50设置", "曲线51设置", "曲线52设置", "曲线53设置", "曲线54设置", "曲线55设置", "曲线56设置", "曲线57设置", "曲线58设置", "曲线59设置", "曲线60设置", "曲线61设置", "曲线62设置", "曲线63设置", "曲线64设置", "ID值", "数据模式"] ("DataInitDef")
                    w328 = T9 4 items=["刷新间隔", "波特率", "布尔1设置项", "布尔2设置项", "布尔3设置项", "布尔4设置项", "布尔5设置项", "布尔6设置项", "布尔7设置项", "布尔8设置项", "显控1设置", "显控2设置", "显控3设置", "显控4设置", "显控5设置", "显控6设置", "显控7设置", "显控8设置", "显控9设置", "显控10设置", "显控11设置", "显控12设置", "设控1设置", "设控2设置", "设控3设置", "设控4设置", "设控5设置", "设控6设置", "设控7设置", "设控8设置", "曲线1设置", "曲线2设置", "曲线3设置", "曲线4设置", "曲线5设置", "曲线6设置", "曲线7设置", "曲线8设置", "曲线9设置", "曲线10设置", "曲线11设置", "曲线12设置", "曲线13设置", "曲线14设置", "曲线15设置", "曲线16设置", "曲线17设置", "曲线18设置", "曲线19设置", "曲线20设置", "曲线21设置", "曲线22设置", "曲线23设置", "曲线24设置", "曲线25设置", "曲线26设置", "曲线27设置", "曲线28设置", "曲线29设置", "曲线30设置", "曲线31设置", "曲线32设置", "曲线33设置", "曲线34设置", "曲线35设置", "曲线36设置", "曲线37设置", "曲线38设置", "曲线39设置", "曲线40设置", "曲线41设置", "曲线42设置", "曲线43设置", "曲线44设置", "曲线45设置", "曲线46设置", "曲线47设置", "曲线48设置", "曲线49设置", "曲线50设置", "曲线51设置", "曲线52设置", "曲线53设置", "曲线54设置", "曲线55设置", "曲线56设置", "曲线57设置", "曲线58设置", "曲线59设置", "曲线60设置", "曲线61设置", "曲线62设置", "曲线63设置", "曲线64设置", "ID值", "数据模式"] ("DataInitDef")
                    w329 = T9 3 items=["刷新间隔", "波特率", "布尔1设置项", "布尔2设置项", "布尔3设置项", "布尔4设置项", "布尔5设置项", "布尔6设置项", "布尔7设置项", "布尔8设置项", "显控1设置", "显控2设置", "显控3设置", "显控4设置", "显控5设置", "显控6设置", "显控7设置", "显控8设置", "显控9设置", "显控10设置", "显控11设置", "显控12设置", "设控1设置", "设控2设置", "设控3设置", "设控4设置", "设控5设置", "设控6设置", "设控7设置", "设控8设置", "曲线1设置", "曲线2设置", "曲线3设置", "曲线4设置", "曲线5设置", "曲线6设置", "曲线7设置", "曲线8设置", "曲线9设置", "曲线10设置", "曲线11设置", "曲线12设置", "曲线13设置", "曲线14设置", "曲线15设置", "曲线16设置", "曲线17设置", "曲线18设置", "曲线19设置", "曲线20设置", "曲线21设置", "曲线22设置", "曲线23设置", "曲线24设置", "曲线25设置", "曲线26设置", "曲线27设置", "曲线28设置", "曲线29设置", "曲线30设置", "曲线31设置", "曲线32设置", "曲线33设置", "曲线34设置", "曲线35设置", "曲线36设置", "曲线37设置", "曲线38设置", "曲线39设置", "曲线40设置", "曲线41设置", "曲线42设置", "曲线43设置", "曲线44设置", "曲线45设置", "曲线46设置", "曲线47设置", "曲线48设置", "曲线49设置", "曲线50设置", "曲线51设置", "曲线52设置", "曲线53设置", "曲线54设置", "曲线55设置", "曲线56设置", "曲线57设置", "曲线58设置", "曲线59设置", "曲线60设置", "曲线61设置", "曲线62设置", "曲线63设置", "曲线64设置", "ID值", "数据模式"] ("DataInitDef")
                    w330 = T9 2 items=["刷新间隔", "波特率", "布尔1设置项", "布尔2设置项", "布尔3设置项", "布尔4设置项", "布尔5设置项", "布尔6设置项", "布尔7设置项", "布尔8设置项", "显控1设置", "显控2设置", "显控3设置", "显控4设置", "显控5设置", "显控6设置", "显控7设置", "显控8设置", "显控9设置", "显控10设置", "显控11设置", "显控12设置", "设控1设置", "设控2设置", "设控3设置", "设控4设置", "设控5设置", "设控6设置", "设控7设置", "设控8设置", "曲线1设置", "曲线2设置", "曲线3设置", "曲线4设置", "曲线5设置", "曲线6设置", "曲线7设置", "曲线8设置", "曲线9设置", "曲线10设置", "曲线11设置", "曲线12设置", "曲线13设置", "曲线14设置", "曲线15设置", "曲线16设置", "曲线17设置", "曲线18设置", "曲线19设置", "曲线20设置", "曲线21设置", "曲线22设置", "曲线23设置", "曲线24设置", "曲线25设置", "曲线26设置", "曲线27设置", "曲线28设置", "曲线29设置", "曲线30设置", "曲线31设置", "曲线32设置", "曲线33设置", "曲线34设置", "曲线35设置", "曲线36设置", "曲线37设置", "曲线38设置", "曲线39设置", "曲线40设置", "曲线41设置", "曲线42设置", "曲线43设置", "曲线44设置", "曲线45设置", "曲线46设置", "曲线47设置", "曲线48设置", "曲线49设置", "曲线50设置", "曲线51设置", "曲线52设置", "曲线53设置", "曲线54设置", "曲线55设置", "曲线56设置", "曲线57设置", "曲线58设置", "曲线59设置", "曲线60设置", "曲线61设置", "曲线62设置", "曲线63设置", "曲线64设置", "ID值", "数据模式"] ("DataInitDef")
                    # "布尔控件状态与表格显示联动"
                    n205 = local write "延时更新布尔状态"(i16 5 ("延时更新布尔状态")) -> ()
                    n206 = local read "控件配置文件"() -> (w296:string[][])
                    n207 = Index Array(array=w296, index (row)=w330, index (col)=1 ("禁用的索引 (列)")) -> (element=w324:string)
                    n208 = Index Array(array=w296, index (row)=w329, index (col)=1 ("禁用的索引 (列)")) -> (element=w320:string)
                    n209 = Index Array(array=w296, index (row)=w328, index (col)=1 ("禁用的索引 (列)")) -> (element=w317:string)
                    n210 = Index Array(array=w296, index (row)=w327, index (col)=1 ("禁用的索引 (列)")) -> (element=w314:string)
                    n211 = Index Array(array=w296, index (row)=w326, index (col)=1 ("禁用的索引 (列)")) -> (element=w311:string)
                    n212 = Index Array(array=w296, index (row)=w310, index (col)=1 ("禁用的索引 (列)")) -> (element=w307:string)
                    n213 = Index Array(array=w296, index (row)=w301, index (col)=1 ("禁用的索引 (列)")) -> (element=w304:string)
                    n214 = Index Array(array=w296, index (row)=w300, index (col)=1 ("禁用的索引 (列)")) -> (element=w297:string)
                    n215 = local read "表格"() -> (w294:string[][])
                    n216 = call "字符串比对X.vi"("字符串"=w324) -> ("布尔"=w325:bool)  [unwired: 10 in]
                    n217 = call "字符串比对X.vi"("字符串"=w311) -> ("布尔"=w312:bool)  [unwired: 10 in]
                    n218 = call "字符串比对X.vi"("字符串"=w307) -> ("布尔"=w306:bool)  [unwired: 10 in]
                    n219 = call "字符串比对X.vi"("字符串"=w320) -> ("布尔"=w321:bool)  [unwired: 10 in]
                    n220 = call "字符串比对X.vi"("字符串"=w314) -> ("布尔"=w315:bool)  [unwired: 10 in]
                    n221 = call "字符串比对X.vi"("字符串"=w304) -> ("布尔"=w305:bool)  [unwired: 10 in]
                    n222 = call "字符串比对X.vi"("字符串"=w297) -> ("布尔"=w295:bool)  [unwired: 10 in]
                    n223 = call "字符串比对X.vi"("字符串"=w317) -> ("布尔"=w318:bool)  [unwired: 10 in]
                    n224 = call "布尔状态识别.vi"("布尔名称"=w324, "表格"=w294, "布尔"=w325) -> ("布尔结果"=w323:bool)  [unwired: 8 in]
                    n225 = call "布尔状态识别.vi"("布尔名称"=w320, "表格"=w294, "布尔"=w321) -> ("布尔结果"=w322:bool)  [unwired: 8 in]
                    n226 = call "布尔状态识别.vi"("布尔名称"=w314, "表格"=w294, "布尔"=w315) -> ("布尔结果"=w316:bool)  [unwired: 8 in]
                    n227 = call "布尔状态识别.vi"("布尔名称"=w311, "表格"=w294, "布尔"=w312) -> ("布尔结果"=w313:bool)  [unwired: 8 in]
                    n228 = call "布尔状态识别.vi"("布尔名称"=w307, "表格"=w294, "布尔"=w306) -> ("布尔结果"=w308:bool)  [unwired: 8 in]
                    n229 = call "布尔状态识别.vi"("布尔名称"=w317, "表格"=w294, "布尔"=w318) -> ("布尔结果"=w319:bool)  [unwired: 8 in]
                    n230 = call "布尔状态识别.vi"("布尔名称"=w304, "表格"=w294, "布尔"=w305) -> ("布尔结果"=w303:bool)  [unwired: 8 in]
                    n231 = call "布尔状态识别.vi"("布尔名称"=w297, "表格"=w294, "布尔"=w295) -> ("布尔结果"=w298:bool)  [unwired: 8 in]
                    n232 = property on="布尔 1" class="Bool (严格)"("Value"=w323) -> ()  [unwired: 2 in, 2 out]
                    n233 = property on="布尔 2" class="Bool (严格)"("Value"=w322) -> ()  [unwired: 2 in, 2 out]
                    n234 = property on="布尔 3" class="Bool (严格)"("Value"=w319) -> ()  [unwired: 2 in, 2 out]
                    n235 = property on="布尔 4" class="Bool (严格)"("Value"=w316) -> ()  [unwired: 2 in, 2 out]
                    n236 = property on="布尔 5" class="Bool (严格)"("Value"=w313) -> ()  [unwired: 2 in, 2 out]
                    n237 = property on="布尔 6" class="Bool (严格)"("Value"=w308) -> ()  [unwired: 2 in, 2 out]
                    n238 = property on="布尔 7" class="Bool (严格)"("Value"=w303) -> ()  [unwired: 2 in, 2 out]
                    n239 = property on="布尔 8" class="Bool (严格)"("Value"=w298) -> ()  [unwired: 2 in, 2 out]
                  }
                }
              }
              event "布尔 1": Value Change {
                w337 = T9 2 items=["刷新间隔", "波特率", "布尔1设置项", "布尔2设置项", "布尔3设置项", "布尔4设置项", "布尔5设置项", "布尔6设置项", "布尔7设置项", "布尔8设置项", "显控1设置", "显控2设置", "显控3设置", "显控4设置", "显控5设置", "显控6设置", "显控7设置", "显控8设置", "显控9设置", "显控10设置", "显控11设置", "显控12设置", "设控1设置", "设控2设置", "设控3设置", "设控4设置", "设控5设置", "设控6设置", "设控7设置", "设控8设置", "曲线1设置", "曲线2设置", "曲线3设置", "曲线4设置", "曲线5设置", "曲线6设置", "曲线7设置", "曲线8设置", "曲线9设置", "曲线10设置", "曲线11设置", "曲线12设置", "曲线13设置", "曲线14设置", "曲线15设置", "曲线16设置", "曲线17设置", "曲线18设置", "曲线19设置", "曲线20设置", "曲线21设置", "曲线22设置", "曲线23设置", "曲线24设置", "曲线25设置", "曲线26设置", "曲线27设置", "曲线28设置", "曲线29设置", "曲线30设置", "曲线31设置", "曲线32设置", "曲线33设置", "曲线34设置", "曲线35设置", "曲线36设置", "曲线37设置", "曲线38设置", "曲线39设置", "曲线40设置", "曲线41设置", "曲线42设置", "曲线43设置", "曲线44设置", "曲线45设置", "曲线46设置", "曲线47设置", "曲线48设置", "曲线49设置", "曲线50设置", "曲线51设置", "曲线52设置", "曲线53设置", "曲线54设置", "曲线55设置", "曲线56设置", "曲线57设置", "曲线58设置", "曲线59设置", "曲线60设置", "曲线61设置", "曲线62设置", "曲线63设置", "曲线64设置", "ID值", "数据模式"] ("DataInitDef")
                n240 = event-data() -> ("NewVal"=w338:bool)  [unwired: 1 in]
                n241 = local read "控件配置文件"() -> (w344:string[][])
                n242 = Index Array(array=w344, index (row)=w337, index (col)=1 ("禁用的索引 (列)")) -> (element=w343:string)
                n243 = Not Equal?(x=w343, y="") -> (x != y?=w340:bool)
                n244 = Not Equal?(x=w343, y="X") -> (x != y?=w339:bool)
                n245 = And(x=w340, y=w339) -> (x .and. y?=w341:bool)
                n246 = case shown="真" w341 {
                  tunnel: w338 -> [_ w359]
                  tunnel: w343 -> [_ w356]
                  frame False {
                  }
                  frame True {
                    n247 = Decimal String To Number(string=w356) -> (number=w349:i32)  [unwired: 2 in, 1 out]
                    n248 = local write "延时更新布尔状态"(i16 0 ("延时更新布尔状态")) -> ()
                    n249 = property on="表格" class="Tbl (严格)"() -> ("Value"=w350:string[][])  [unwired: 2 in, 2 out]
                    n250 = Index Array(array=w350, index (row)=w349, index (col)=7 ("禁用的索引 (列)")) -> (element=w348:string)
                    n251 = Index Array(array=w350, index (row)=w349, index (col)=1 ("禁用的索引 (列)")) -> (element=w355:string)
                    n252 = Hexadecimal String To Number(string=w348) -> (number=w347:u32)  [unwired: 2 in, 1 out]
                    n253 = Decimal String To Number(string=w355) -> (number=w353:i32)  [unwired: 2 in, 1 out]
                    n254 = To Unsigned Word Integer(number=w353) -> (unsigned 16bit integer=w360:u16)
                    n255 = Boolean To (0,1)(Boolean=w359) -> (0, 1=w358:i16)
                    n256 = Bundle(w360, w358, w349, w347) -> (w357:cluster{u16, i16, i32, u32})  [unwired: 1 in]
                    n257 = property on="要发送的数据" class="Clust (严格)"("Val(Sgnl)"=w357) -> ()  [unwired: 2 in, 2 out]
                  }
                }
              }
              event "设控1": Value Change {
                w361 = T9 22 items=["刷新间隔", "波特率", "布尔1设置项", "布尔2设置项", "布尔3设置项", "布尔4设置项", "布尔5设置项", "布尔6设置项", "布尔7设置项", "布尔8设置项", "显控1设置", "显控2设置", "显控3设置", "显控4设置", "显控5设置", "显控6设置", "显控7设置", "显控8设置", "显控9设置", "显控10设置", "显控11设置", "显控12设置", "设控1设置", "设控2设置", "设控3设置", "设控4设置", "设控5设置", "设控6设置", "设控7设置", "设控8设置", "曲线1设置", "曲线2设置", "曲线3设置", "曲线4设置", "曲线5设置", "曲线6设置", "曲线7设置", "曲线8设置", "曲线9设置", "曲线10设置", "曲线11设置", "曲线12设置", "曲线13设置", "曲线14设置", "曲线15设置", "曲线16设置", "曲线17设置", "曲线18设置", "曲线19设置", "曲线20设置", "曲线21设置", "曲线22设置", "曲线23设置", "曲线24设置", "曲线25设置", "曲线26设置", "曲线27设置", "曲线28设置", "曲线29设置", "曲线30设置", "曲线31设置", "曲线32设置", "曲线33设置", "曲线34设置", "曲线35设置", "曲线36设置", "曲线37设置", "曲线38设置", "曲线39设置", "曲线40设置", "曲线41设置", "曲线42设置", "曲线43设置", "曲线44设置", "曲线45设置", "曲线46设置", "曲线47设置", "曲线48设置", "曲线49设置", "曲线50设置", "曲线51设置", "曲线52设置", "曲线53设置", "曲线54设置", "曲线55设置", "曲线56设置", "曲线57设置", "曲线58设置", "曲线59设置", "曲线60设置", "曲线61设置", "曲线62设置", "曲线63设置", "曲线64设置", "ID值", "数据模式"] ("DataInitDef")
                n258 = event-data() -> ("NewVal"=w365:string)  [unwired: 1 in, 5 out]
